vi "CRYAPI WSYSTEM LIB.vi"(8 "tFrame":T4, 9 "sData":string, 10 "nData":i32, 11 "sAction":string) -> (0 "nData_Out":i32, 1 "sData_Out":string, 3 "tFrame_Out":T4)   [LabVIEW 2013]
uses:
  <vilib>/Utility/miscctls.llb/LVRectTypeDef.ctl
  CRYMain Sub Window Global.vi
panel:
  in  "sOption":string
  in  "tSpliterSave":T2
  in  "cWinStatus":cluster{"nData":i32, "nActiveNum":i32}[](array[cluster])
  in  "nSpliterPos":T3(array[cluster])
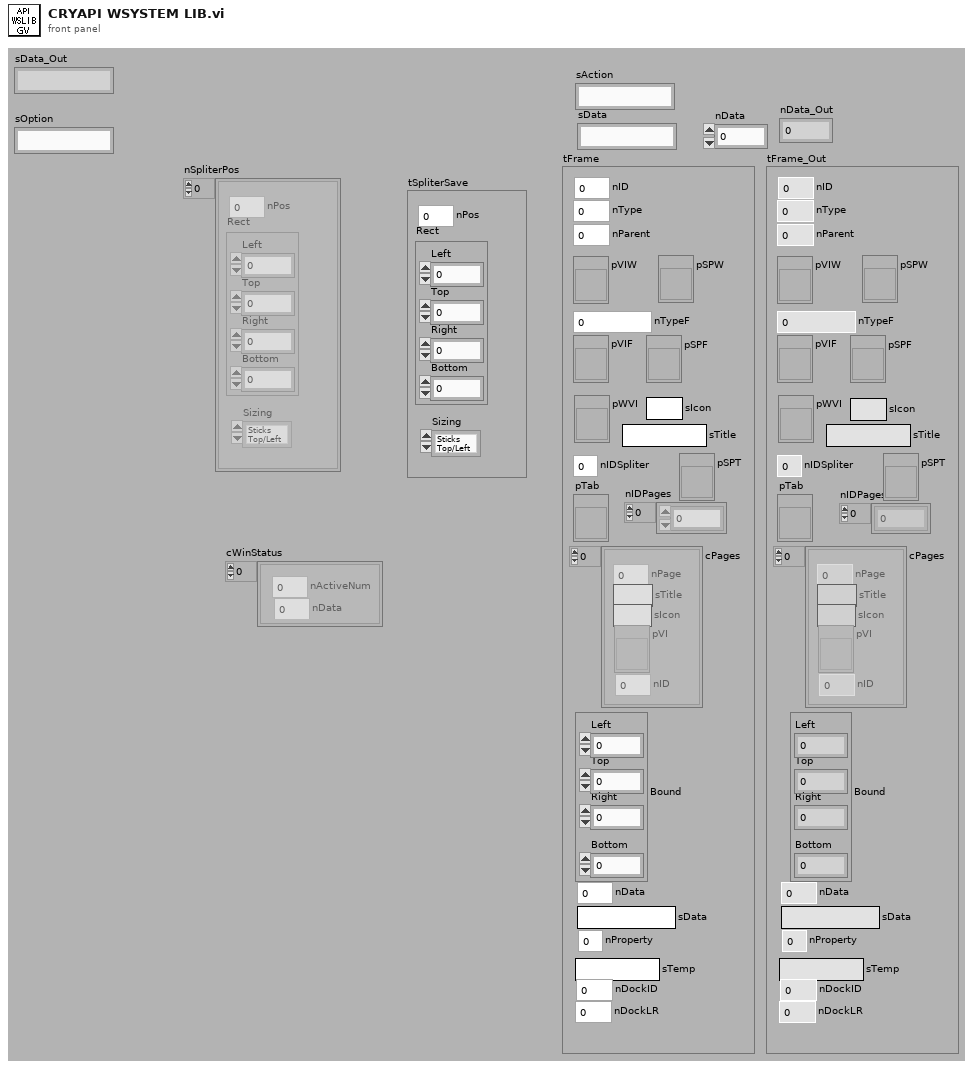
[diagram p1: front panel]
types:
  T1 = typedef "LVRectTypeDef.ctl" = cluster{"Left":i16, "Top":i16, "Right":i16, "Bottom":i16}
  T2 = cluster{"nPos":i32, "Rect":T1, "Sizing":enum16{"Sticks Top/Left", "Sticks Bottom/Right", "Proportional"}}
  T3 = cluster{"nPos":i32, "Rect":T1, "Sizing":enum16{"Sticks Top/Left", "Sticks Bottom/Right", "Proportional"}}[]
  T4 = cluster{"nType":i32, "nParent":i32, "pVIW":refnum<vi>, "pSPW":refnum<vi>, "nTypeF":i32, "pVIF":refnum<vi>, "pSPF":refnum<vi>, "nIDSpliter":i32, "nProperty":i32, "Bound":T1, "nID":i32, "nData":i32, "sData":string, "pWVI":refnum<vi>, "sTitle":string, "cPages":cluster{"nPage":i32, "sTitle":string, "sIcon":string, "pVI":refnum<vi>, "nID":i32}[], "pTab":refnum<vi>, "nIDPages":i32[], "pSPT":refnum<vi>, "sTemp":string, "nDockID":i32, "nDockLR":i32, "sIcon":string}
  T5 = cluster{"nID":i32[], "Frame":cluster{"nType":i32, "nParent":i32, "pVIW":refnum<vi>, "pSPW":refnum<vi>, "nTypeF":i32, "pVIF":refnum<vi>, "pSPF":refnum<vi>, "nIDSpliter":i32, "nProperty":i32, "Bound":T1, "nID":i32, "nData":i32, "sData":string, "pWVI":refnum<vi>, "sTitle":string, "cPages":cluster{"nPage":i32, "sTitle":string, "sIcon":string, "pVI":refnum<vi>, "nID":i32}[], "pTab":refnum<vi>, "nIDPages":i32[], "pSPT":refnum<vi>, "sTemp":string, "nDockID":i32, "nDockLR":i32, "sIcon":string}[]}
  T6 = cluster{"nPage":i32, "sTitle":string, "sIcon":string, "pVI":refnum<vi>, "nID":i32}
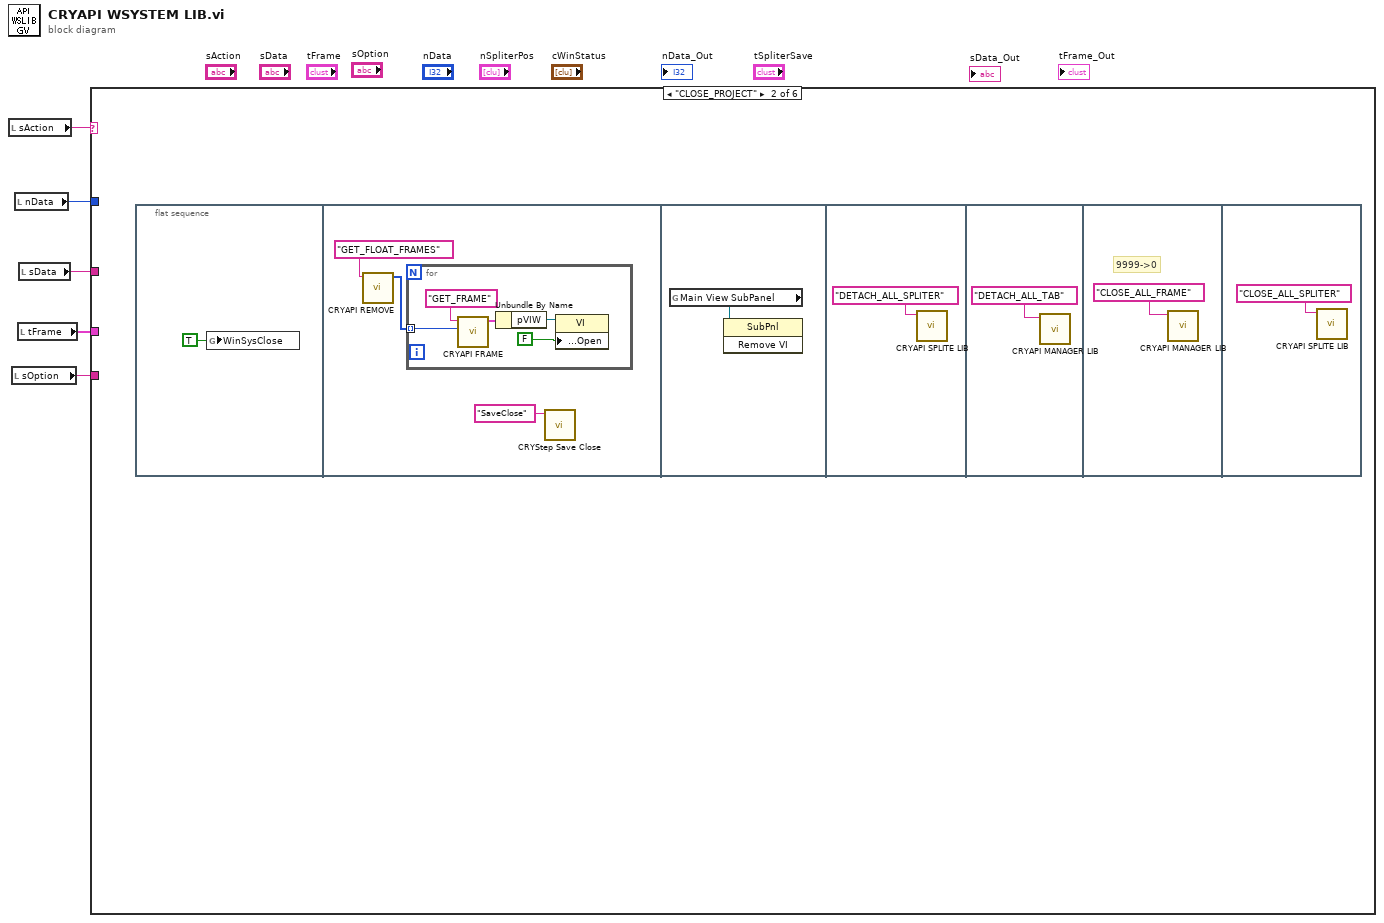
[diagram p0: block diagram]
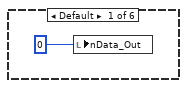
[diagram p2: hidden frame]
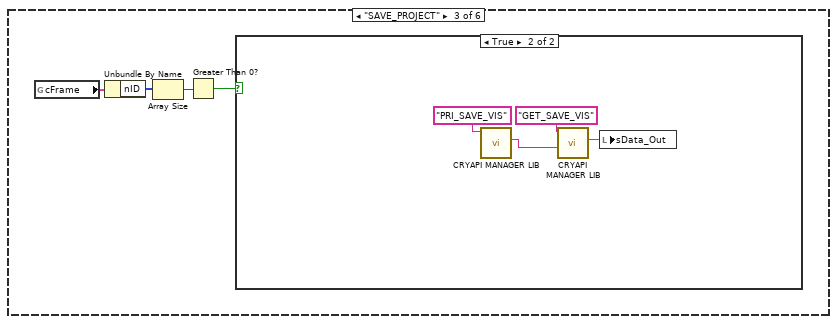
[diagram p3: hidden frame]
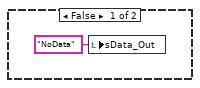
[diagram p4: hidden frame]
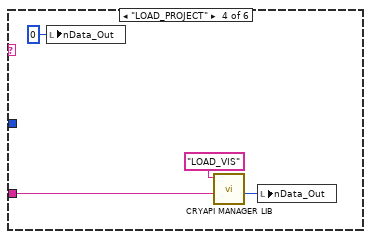
[diagram p5: hidden frame]
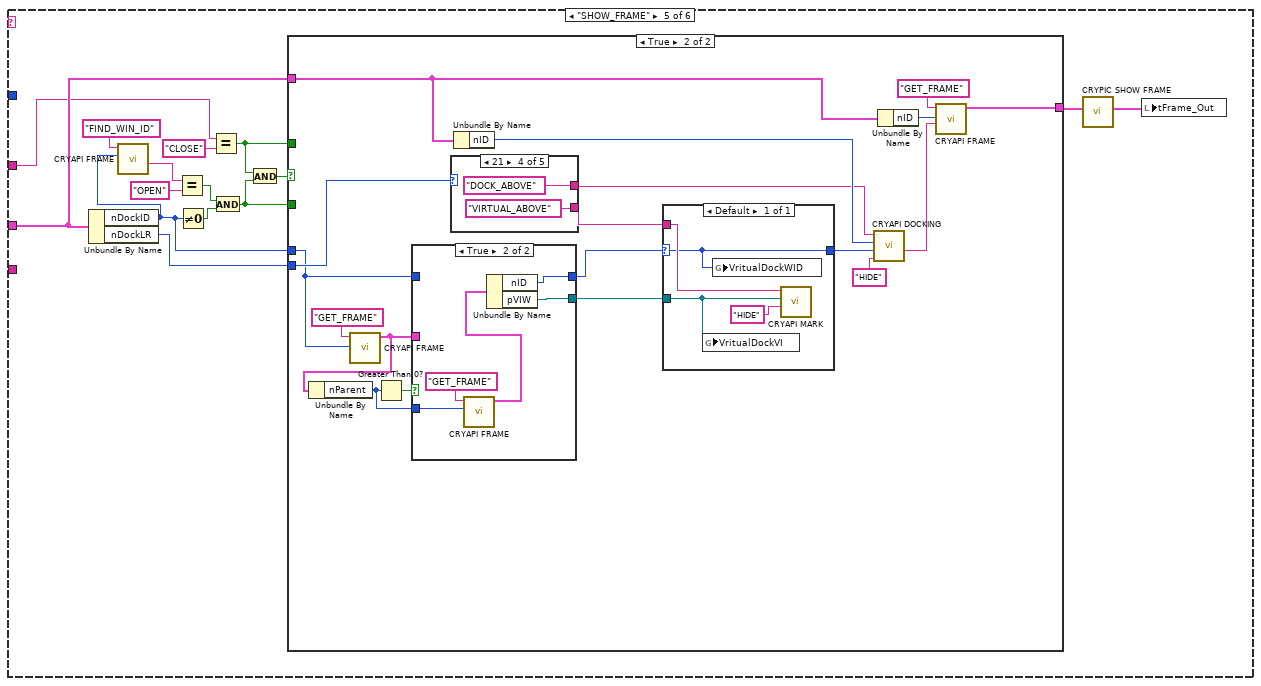
[diagram p6: hidden frame]
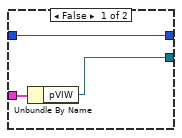
[diagram p8: hidden frame]
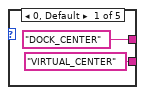
[diagram p9: hidden frame]
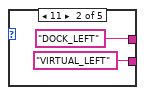
[diagram p10: hidden frame]
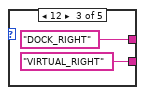
[diagram p11: hidden frame]
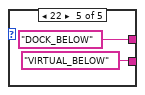
[diagram p12: hidden frame]
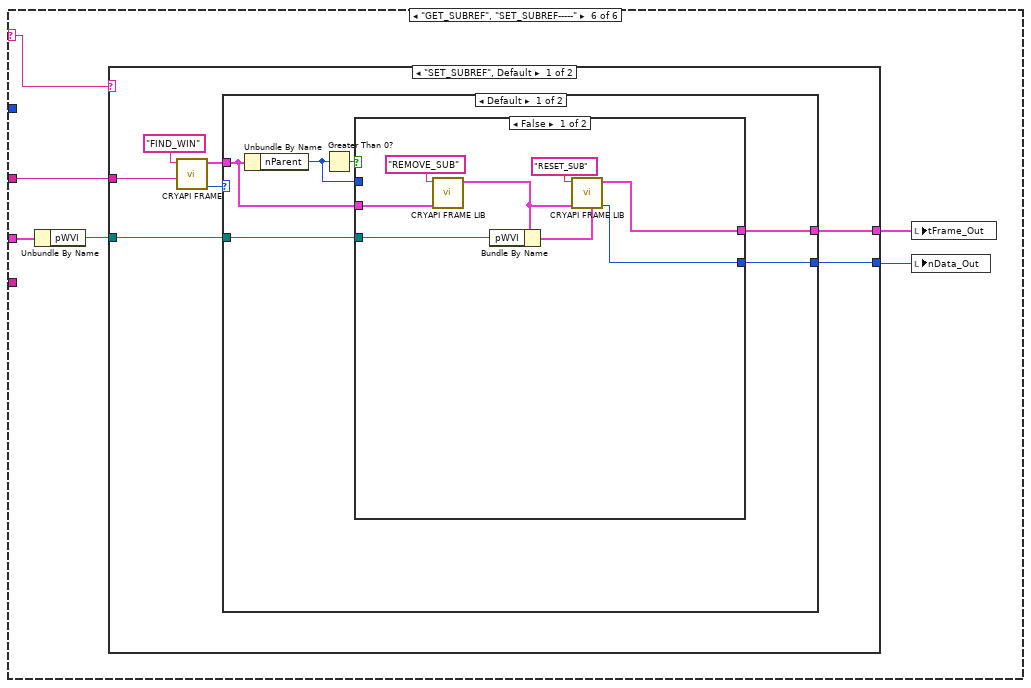
[diagram p13: hidden frame]
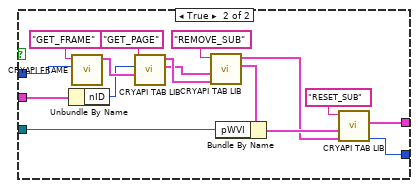
[diagram p14: hidden frame]
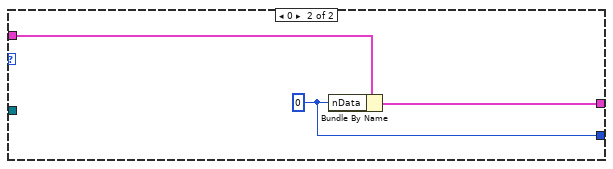
[diagram p15: hidden frame]
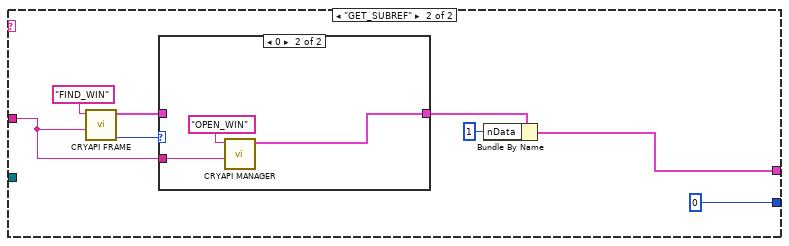
[diagram p16: hidden frame]
diagram:
  n1 = local read "sAction"() -> (w5:string)
  n2 = local read "sOption"() -> (w1:string)
  n3 = local read "nData"() -> (w3:i32)
  n4 = local read "tFrame"() -> (w2:T4)
  n5 = local read "sData"() -> (w4:string)
  n6 = case shown="\"CLOSE_PROJECT\"" w5 {
    selector: w5 -> [_ _ _ _ _ w95]
    tunnel: w4 -> [_ _ _ w30 w39 w94]
    tunnel: w3 -> [_ _ _ _ _ _]
    tunnel: w2 -> [_ _ _ _ w48 w93]
    tunnel: w1 -> [_ _ _ _ _ _]
    frame Default {
      n7 = local write "nData_Out"(0 ("nData_Out")) -> ()
    }
    frame "CLOSE_PROJECT" {
      n8 = flat-sequence {
        frame #0 {
          n9 = global write "CRYMain Sub Window Global.vi" "WinSysClose"(TRUE ("WinSysClose")) -> ()
        }
        frame #1 {
          n10 = call "CRYAPI REMOVE.vi"("sAction"="GET_FLOAT_FRAMES") -> ("List_ID_Out"=w9:i32[])  [unwired: 4 in, 6 out]
          n11 = for {
            tunnel: w9 -> [w15] mode=indexing
            n12 = call "CRYAPI FRAME.vi"("nData"=w15, "sAction"="GET_FRAME") -> ("tFrame_Out"=w13:T4)  [unwired: 4 in, 5 out]
            n13 = Unbundle By Name(w13) -> ("pVIW"=w11:refnum<vi>)
            n14 = property class="VI"(reference=w11, "Front Panel.Open"=FALSE ("Visible")) -> ()  [unwired: 1 in, 2 out]
          }
          n15 = call "CRYStep Save Close.vi"("sAction"="SaveClose") -> ()  [unwired: 11 in]
        }
        frame #2 {
          n16 = global read "CRYMain Sub Window Global.vi" "Main View SubPanel"() -> (w16:refnum<vi>)
          n17 = invoke class="SubPnl" method="Remove VI"(reference=w16) -> ()  [unwired: 2 in, 3 out]
        }
        frame #3 {
          n18 = call "CRYAPI SPLITE LIB.vi"("sAction"="DETACH_ALL_SPLITER") -> ()  [unwired: 8 in, 3 out]
        }
        frame #4 {
          n19 = call "CRYAPI MANAGER LIB.vi"("sAction"="DETACH_ALL_TAB") -> ()  [unwired: 8 in, 3 out]
        }
        frame #5 {
          # "9999->0"
          n20 = call "CRYAPI MANAGER LIB.vi"("sAction"="CLOSE_ALL_FRAME") -> ()  [unwired: 8 in, 3 out]
        }
        frame #6 {
          n21 = call "CRYAPI SPLITE LIB.vi"("sAction"="CLOSE_ALL_SPLITER") -> ()  [unwired: 8 in, 3 out]
        }
      }
    }
    frame "SAVE_PROJECT" {
      n22 = global read "CRYMain Sub Window Global.vi" "cFrame"() -> (w22:T5)
      n23 = Unbundle By Name(w22) -> ("nID"=w21:i32[])
      n24 = Array Size(array=w21) -> (size(s)=w23:i32)
      n25 = Greater Than 0?(x=w23) -> (x > 0?=w24:bool)
      n26 = case shown="True" w24 {
        frame False {
          n27 = local write "sData_Out"("NoData" ("sData_Out")) -> ()
        }
        frame True {
          n28 = call "CRYAPI MANAGER LIB.vi"("sAction"="PRI_SAVE_VIS") -> ("sData_Out"=w26:string)  [unwired: 4 in, 6 out]
          n29 = call "CRYAPI MANAGER LIB.vi"("sData"=w26, "sAction"="GET_SAVE_VIS") -> ("sData_Out"=w28:string)  [unwired: 3 in, 6 out]
          n30 = local write "sData_Out"(w28) -> ()
        }
      }
    }
    frame "LOAD_PROJECT" {
      n31 = local write "nData_Out"(0 ("nData_Out")) -> ()
      n32 = call "CRYAPI MANAGER LIB.vi"("sData"=w30, "sAction"="LOAD_VIS") -> ("nData_Out"=w31:i32)  [unwired: 3 in, 6 out]
      n33 = local write "nData_Out"(w31) -> ()
    }
    frame "SHOW_FRAME" {
      n34 = Unbundle By Name(w48) -> ("nDockID"=w43:i32, "nDockLR"=w46:i32)
      n35 = call "CRYAPI FRAME.vi"("nData"=w43, "sAction"="FIND_WIN_ID") -> ("sData_Out"=w42:string)  [unwired: 4 in, 5 out]
      n36 = Equal?(x=w42, y="OPEN") -> (x = y?=w40:bool)
      n37 = Not Equal To 0?(x=w43) -> (x != 0?=w45:bool)
      n38 = Equal?(x=w39, y="CLOSE") -> (x = y?=w38:bool)
      n39 = And(x=w40, y=w45) -> (x .and. y?=w37:bool)
      n40 = And(x=w38, y=w37) -> (x .and. y?=w34:bool)
      n41 = case shown="True" w34 {
        tunnel: w48 -> [w49 w59]
        tunnel: [w49 w50] -> w36
        tunnel: w46 -> [_ w67]
        tunnel: w43 -> [_ w55]
        tunnel: w38 -> [_ _]
        tunnel: w37 -> [_ _]
        frame False {
        }
        frame True {
          n42 = call "CRYAPI FRAME.vi"("nData"=w55, "sAction"="GET_FRAME") -> ("tFrame_Out"=w53:T4)  [unwired: 4 in, 5 out]
          n43 = Unbundle By Name(w53) -> ("nParent"=w51:i32)
          n44 = Greater Than 0?(x=w51) -> (x > 0?=w52:bool)
          n45 = case shown="True" w52 {
            tunnel: w53 -> [w69 _]
            tunnel: [w68 w75] -> w56
            tunnel: w55 -> [w70 _]
            tunnel: [w70 w72] -> w54
            tunnel: w51 -> [_ w73]
            frame False {
              n46 = Unbundle By Name(w69) -> ("pVIW"=w68:refnum<vi>)
            }
            frame True {
              n47 = call "CRYAPI FRAME.vi"("nData"=w73, "sAction"="GET_FRAME") -> ("tFrame_Out"=w71:T4)  [unwired: 4 in, 5 out]
              n48 = Unbundle By Name(w71) -> ("nID"=w72:i32, "pVIW"=w75:refnum<vi>)
            }
          }
          n49 = case shown="21" w67 {
            tunnel: ["DOCK_CENTER" ("sAction") "DOCK_LEFT" ("sAction") "DOCK_RIGHT" ("sAction") "DOCK_ABOVE" ("sAction") "DOCK_BELOW" ("sAction")] -> w64
            tunnel: ["VIRTUAL_CENTER" "VIRTUAL_LEFT" "VIRTUAL_RIGHT" "VIRTUAL_ABOVE" "VIRTUAL_BELOW"] -> w63
            frame 0, Default {
            }
            frame 11 {
            }
            frame 12 {
            }
            frame 21 {
            }
            frame 22 {
            }
          }
          n50 = Unbundle By Name(w59) -> ("nID"=w65:i32)
          n51 = case shown="Default" w54 {
            selector: w54 -> [w76]
            tunnel: [w76] -> w62
            tunnel: w56 -> [w78]
            tunnel: w63 -> [w77]
            frame Default {
              n52 = global write "CRYMain Sub Window Global.vi" "VritualDockVI"(w78) -> ()
              n53 = global write "CRYMain Sub Window Global.vi" "VritualDockWID"(w76) -> ()
              n54 = call "CRYAPI MARK.vi"("sAction"=w77, "mVritual_VIRef"=w78, "sData"="HIDE") -> ()  [unwired: 1 in, 7 out]
            }
          }
          n55 = call "CRYAPI DOCKING.vi"("sData"="HIDE", "nDWinID"=w62, "nSWinID"=w65, "sAction"=w64) -> ("sData_Out"=w58:string)  [unwired: 7 out]
          n56 = Unbundle By Name(w59) -> ("nID"=w60:i32)
          n57 = call "CRYAPI FRAME.vi"("sData"=w58, "nData"=w60, "sAction"="GET_FRAME") -> ("tFrame_Out"=w50:T4)  [unwired: 3 in, 5 out]
        }
      }
      n58 = call "CRYPIC SHOW FRAME.vi"("tFrame"=w36) -> ("tFrame_Out"=w35:T4)  [unwired: 10 in]
      n59 = local write "tFrame_Out"(w35) -> ()
    }
    frame "GET_SUBREF", "SET_SUBREF-----" {
      n60 = Unbundle By Name(w93) -> ("pWVI"=w92:refnum<vi>)
      n61 = case shown="\"SET_SUBREF\", Default" w95 {
        tunnel: w94 -> [w101 w140]
        tunnel: w92 -> [w98 _]
        tunnel: [w97 w137] -> w91
        tunnel: [w96 0 ("nData")] -> w90
        frame "SET_SUBREF", Default {
          n62 = call "CRYAPI FRAME.vi"("sData"=w101, "sAction"="FIND_WIN") -> ("nData_Out"=w100:i32, "tFrame_Out"=w99:T4)  [unwired: 4 in, 4 out]
          n63 = case shown="Default" w100 {
            tunnel: w99 -> [w104 w135]
            tunnel: w98 -> [w106 _]
            tunnel: [w105 w134] -> w97
            tunnel: [w103 w133] -> w96
            frame Default {
              n64 = Unbundle By Name(w104) -> ("nParent"=w107:i32)
              n65 = Greater Than 0?(x=w107) -> (x > 0?=w108:bool)
              n66 = case shown="False" w108 {
                tunnel: w107 -> [_ w131]
                tunnel: w106 -> [w115 w128]
                tunnel: [w113 w121] -> w105
                tunnel: w104 -> [w112 w119]
                tunnel: [w109 w117] -> w103
                frame False {
                  n67 = call "CRYAPI FRAME LIB.vi"("tFrame"=w112, "sAction"="REMOVE_SUB") -> ("tFrame_Out"=w110:T4)  [unwired: 4 in, 5 out]
                  n68 = Bundle By Name(cluster=w110, "pWVI"=w115) -> (w111:T4)
                  n69 = call "CRYAPI FRAME LIB.vi"("tFrame_In"=w111, "tFrame"=w110, "sAction"="RESET_SUB") -> ("nData_Out"=w109:i32, "tFrame_Out"=w113:T4)  [unwired: 3 in, 4 out]
                }
                frame True {
                  n70 = Unbundle By Name(w119) -> ("nID"=w118:i32)
                  n71 = call "CRYAPI FRAME.vi"("nData"=w131, "sAction"="GET_FRAME") -> ("tFrame_Out"=w124:T4)  [unwired: 4 in, 5 out]
                  n72 = call "CRYAPI TAB LIB.vi"("tFrame"=w124, "nData"=w118, "sAction"="GET_PAGE") -> ("tFrame_Out"=w122:T4, "tPage_Out"=w123:T6)  [unwired: 1 in, 6 out]
                  n73 = call "CRYAPI TAB LIB.vi"("tPage"=w123, "tFrame"=w122, "sAction"="REMOVE_SUB") -> ("tFrame_Out"=w129:T4, "tPage_Out"=w120:T6)  [unwired: 1 in, 6 out]
                  n74 = Bundle By Name(cluster=w129, "pWVI"=w128) -> (w126:T4)
                  n75 = call "CRYAPI TAB LIB.vi"("tPage"=w120, "tFrame"=w126, "sAction"="RESET_SUB") -> ("nData_Out"=w117:i32, "tFrame_Out"=w121:T4)  [unwired: 1 in, 6 out]
                }
              }
            }
            frame 0 {
              w133 = 0 ("nData")
              n76 = Bundle By Name(cluster=w135, "nData"=w133) -> (w134:T4)
            }
          }
        }
        frame "GET_SUBREF" {
          n77 = call "CRYAPI FRAME.vi"("sData"=w140, "sAction"="FIND_WIN") -> ("nData_Out"=w142:i32, "tFrame_Out"=w141:T4)  [unwired: 4 in, 4 out]
          n78 = case shown="0" w142 {
            tunnel: w141 -> [w144 _]
            tunnel: [w144 w145] -> w139
            tunnel: w140 -> [_ w147]
            frame Default {
            }
            frame 0 {
              n79 = call "CRYAPI MANAGER.vi"("sData"=w147, "sAction"="OPEN_WIN") -> ("tFrame_Out"=w145:T4)  [unwired: 3 in, 6 out]
            }
          }
          n80 = Bundle By Name(cluster=w139, "nData"=1) -> (w137:T4)
        }
      }
      n81 = local write "tFrame_Out"(w91) -> ()
      n82 = local write "nData_Out"(w90) -> ()
    }
  }
